vi "Read Calibration Values.vi"(8 "error in (no error)":errorcluster, 11 "HTS221 in":refnum<class "HTS221.lvclass">) -> (0 "error out":errorcluster, 3 "HTS221 out":refnum<class "HTS221.lvclass">)   [LabVIEW 2020, in "HTS221.lvclass"]
doc: "Reads and stores the temperature and humidity calibration values from the HTS221 device."
uses:
  HTS221.lvclass
  HTS221.lvclass/HTS221.ctl
  Write Humidity.Slope.vi
  Write Humidity.Zero.vi
  Write Temperature.Slope.vi
  Write Temperature.Zero.vi
  LINX I2C/LINX I2C.lvclass
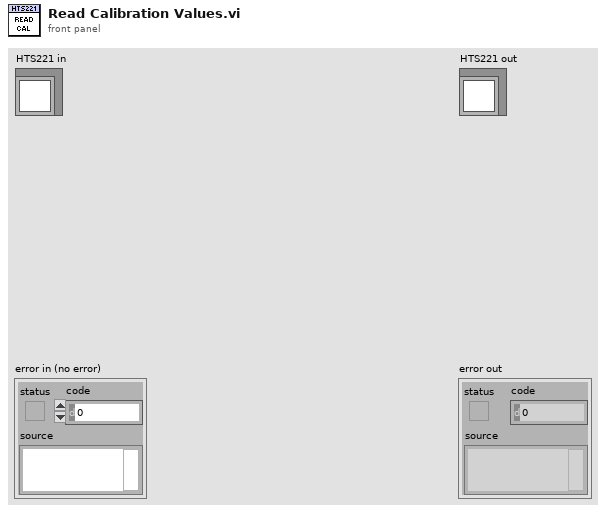
[diagram p1: front panel]
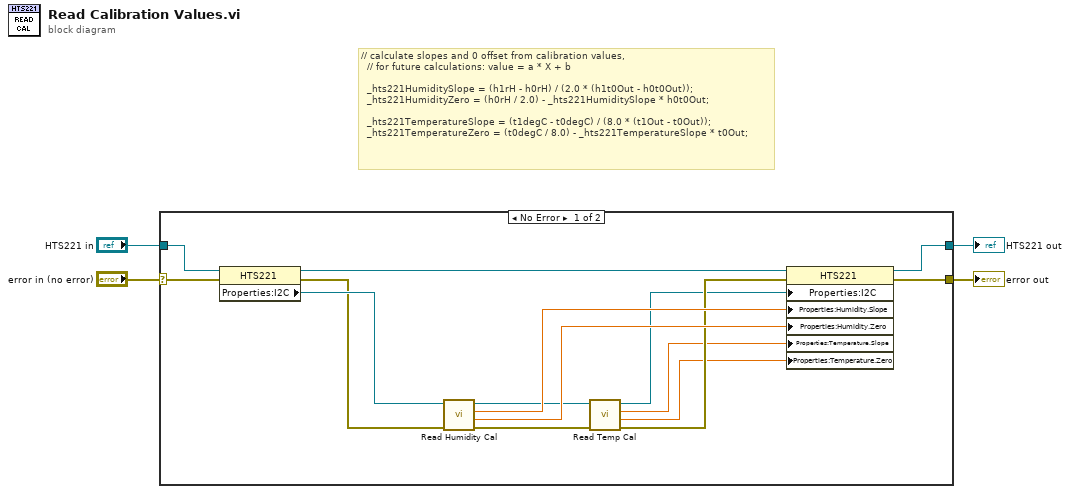
[diagram p0: block diagram]
diagram:
  # "// calculate slopes and 0 offset from calibration values,\n  // for future calculations: value = a * X + b\n\n  _hts221HumiditySlope = (h1rH - h0rH) / (2.0 * (h1t0Out - h0t0Out));\n  _hts221HumidityZero = (h0rH / 2.0) - _hts221HumiditySlope * h0t0Out;\n\n  _hts221TemperatureSlope = (t1degC - t0degC) / (8.0 * (t1Out - t0Out));\n  _hts221TemperatureZero = (t0degC / 8.0) - _hts221TemperatureSlope * t0Out;"
  n1 = case shown="No Error" "error in (no error)" {
    selector: "error in (no error)" -> [w16 w21]
    tunnel: [w14 w21] -> w3
    tunnel: [w15 w20] -> w1
    tunnel: "HTS221 in" -> [w19 w20]
    frame No Error {
      n2 = property class="HTS221"(reference=w19, error in=w16) -> (reference out=w18:refnum<class "HTS221.lvclass">, error out=w13:errorcluster, "Properties:I2C"=w17:refnum<class "LINX I2C.lvclass">)
      n3 = call "Read Humidity Cal.vi"("error in (no error)"=w13, "LINX I2C in"=w17) -> ("error out"=w10:errorcluster, "Zero"=w11:dbl, "Slope"=w12:dbl, "LINX I2C out"=w8:refnum<class "LINX I2C.lvclass">)  [unwired: 6 in]
      n4 = call "Read Temp Cal.vi"("error in (no error)"=w10, "LINX I2C in"=w8) -> ("error out"=w9:errorcluster, "Zero"=w5:dbl, "Slope"=w6:dbl, "LINX I2C out"=w7:refnum<class "LINX I2C.lvclass">)  [unwired: 6 in]
      n5 = property class="HTS221"(reference=w18, error in=w9, "Properties:I2C"=w7, "Properties:Humidity.Slope"=w12, "Properties:Humidity.Zero"=w11, "Properties:Temperature.Slope"=w6, "Properties:Temperature.Zero"=w5) -> (reference out=w15:refnum<class "HTS221.lvclass">, error out=w14:errorcluster)
    }
    frame Error {
    }
  }
  "error out" <- w3
  "HTS221 out" <- w1
